vi "Read Version.vi"(8 "error in (no error)":errorcluster, 11 "DeployResource in":refnum<class "DeployResource.lvclass">) -> (0 "error out":errorcluster, 1 "Build":timestamp, 2 "Version":string, 3 "DeployResource out":refnum<class "DeployResource.lvclass">)   [LabVIEW 2020, in "PicoG-Core.lvlib" / "DeployResource.lvclass"]
uses:
  DeployResource.lvclass
  PicoG-Core.lvlib
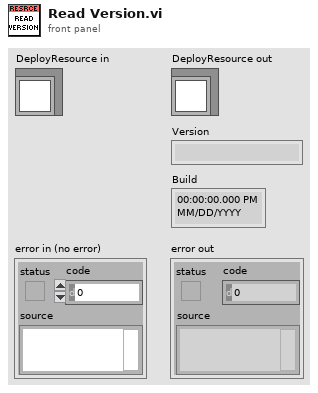
[diagram p1: front panel]
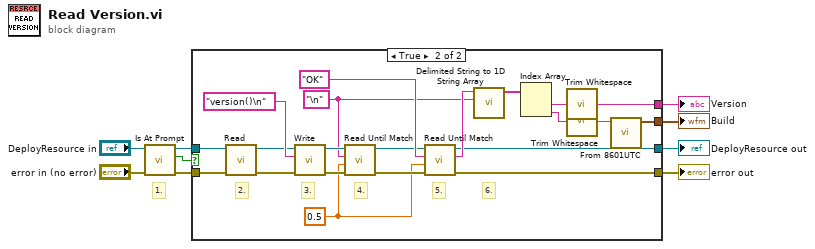
[diagram p0: block diagram]
diagram:
  # "1."
  n1 = call-dynamic "Is At Prompt.vi"("error in (no error)"="error in (no error)", "DeployResource in"="DeployResource in") -> ("error out"=w5:errorcluster, "At Prompt?"=w7:bool, "DeployResource out"=w6:refnum<class "DeployResource.lvclass">)  [unwired: 6 in, 1 out]
  n2 = case shown="True" w7 {
    tunnel: w6 -> [w11 w31]
    tunnel: w5 -> [w10 w30]
    tunnel: [w11 w24] -> w4
    tunnel: [w10 w23] -> w3
    tunnel: [_ w15] -> w2
    tunnel: [_ w12] -> w1
    frame False {
      # "#ERROR"
    }
    frame True {
      w16 = 0.5 ("Timeout S (0)")
      w17 = "\n" ("Data")
      # "6."
      # "5."
      # "4."
      # "3."
      # "2."
      n3 = call "Read.vi"("error in (no error)"=w30, "DeployResource in"=w31) -> ("error out"=w28:errorcluster, "DeployResource out"=w29:refnum<class "DeployResource.lvclass">)  [unwired: 6 in, 2 out]
      n4 = call "Write.vi"("error in (no error)"=w28, "Data"="version()\n", "DeployResource in"=w29) -> ("error out"=w20:errorcluster, "DeployResource out"=w21:refnum<class "DeployResource.lvclass">)  [unwired: 6 in, 1 out]
      n5 = call "Read Until Match.vi"("error in (no error)"=w20, "Timeout S (0)"=w16, "Match String"=w17, "DeployResource in"=w21) -> ("error out"=w18:errorcluster, "DeployResource out"=w19:refnum<class "DeployResource.lvclass">)  [unwired: 4 in, 2 out]
      n6 = call "Read Until Match.vi"("error in (no error)"=w18, "Timeout S (0)"=w16, "Match String"="OK" ("Data"), "DeployResource in"=w19) -> ("error out"=w23:errorcluster, "Data"=w27:string, "DeployResource out"=w24:refnum<class "DeployResource.lvclass">)  [unwired: 4 in, 1 out]
      n7 = call <vilib>:"Delimited String to 1D String Array.vi"("delimiter"=w17, "delimited string"=w27) -> ("string array"=w26:string[])  [unwired: 9 in]
      n8 = Index Array(array=w26) -> (element #1=w25:string, element #2=w14:string)  [unwired: 2 in]
      n9 = call <vilib>:"Trim Whitespace.vi"("string"=w25) -> ("trimmed string"=w15:string)  [unwired: 1 in]
      n10 = call <vilib>:"Trim Whitespace.vi"("string"=w14) -> ("trimmed string"=w13:string)  [unwired: 1 in]
      n11 = call "From 8601UTC.vi"("ISO-8601"=w13) -> ("time stamp"=w12:timestamp)  [unwired: 9 in, 1 out]
    }
  }
  "error out" <- w3
  "DeployResource out" <- w4
  "Version" <- w2
  "Build" <- w1
